vi "Build Blackboard Tag Table.vi"(8 "error in (no error)":errorcluster, 11 "Blackboard in":refnum<class "Blackboard.lvclass">) -> (0 "error out":errorcluster, 1 "Values":refnum<class "Abs_Value.lvclass">[](array[class]), 2 "Table":string[][](array[string]), 3 "Blackboard out":refnum<class "Blackboard.lvclass">)   [LabVIEW 2021]
uses:
  Blackboard/Blackboard.lvclass
  <vilib>/TSA/Abstract Data Classes/Abs_Types/Value/Abs_Value.lvclass
  <vilib>/TSA/Abstract Data Classes/Abs_Types/Integer/Abs_Integer.lvclass
  C:/Program Files (x86)/National Instruments/LabVIEW 2021/vi.lib/TSA/Abstract Data Classes/Abs_Types/Numeric/Abs_Numeric.lvclass
  C:/Program Files (x86)/National Instruments/LabVIEW 2021/vi.lib/TSA/Abstract Data Classes/Abs_Types/Value/Abs_Value.lvclass
  C:/Program Files (x86)/National Instruments/LabVIEW 2021/vi.lib/TSA/Abstract Data Classes/Abs_Types/Type/Abs_Type.lvclass
  C:/Program Files (x86)/National Instruments/LabVIEW 2021/vi.lib/TSA/Abstract Data Classes/Abs_Types/Integer/Abs_Integer.lvclass
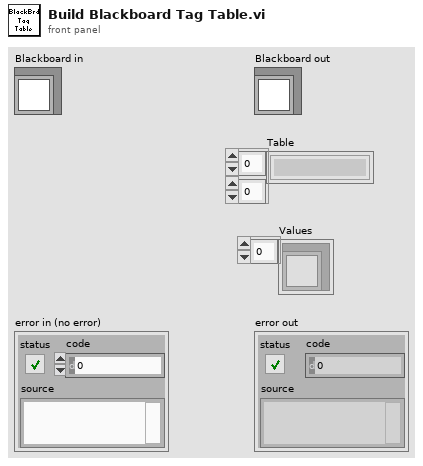
[diagram p1: front panel]
types:
  T1 = typedef "NI_Data Type.lvlib/Data Type.ctl" = enum8{"Invalid Type", "Void", "I8", "I16", "I32", "I64", "U8", "U16", "U32", "U64", "Single Float", "Double Float", "Extended Float", "Single Complex", "Double Complex", "Extended Complex", "Enum U8", "Enum U16", "Enum U32", "Enum U64", "Single Float With Unit", "Double Float With Unit", "Extended Float With Unit", "Single Complex with Unit", "Double Complex with Unit", "Extended Complex with Unit", "Boolean", "String", "Path", "Picture", "Tag", "Array", "Cluster", "Variant", "LV Variant", "Waveform", "Timestamp", "Digital Waveform", "Digital Data", "ExpressData", "Refnum", "External Data", "VI", "Poly VI", "LabVIEW Class Instance", "Fixed Point", "Set Collection", "Map Collection"}
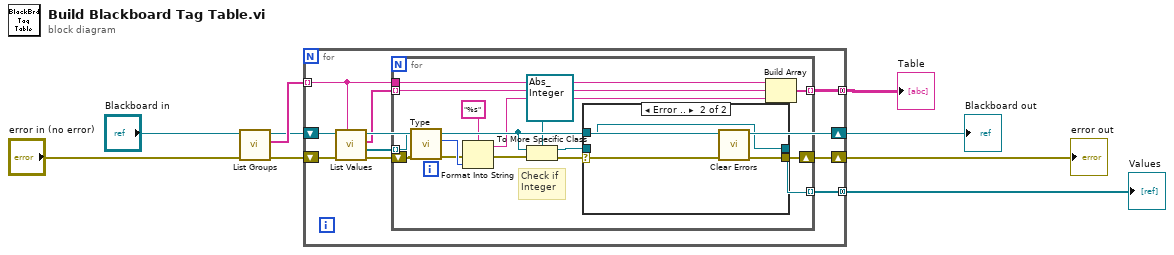
[diagram p0: block diagram]
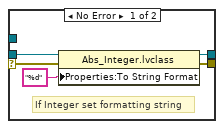
[diagram p2: hidden frame]
diagram:
  n1 = call "List Groups.vi"("error in (no error)"="error in (no error)", "Blackboard in"="Blackboard in") -> ("error out"=w6:errorcluster, "Groups"=w7:string[], "Blackboard out"=w4:refnum<class "Blackboard.lvclass">)  [unwired: 7 in]
  n2 = for {
    shift-right: [w19] -> w3
    shift-left: w4 -> [w18]
    shift-right: [w11] -> w2
    shift-left: w6 -> [w17]
    tunnel: w7 -> [w16] mode=indexing
    tunnel: [w14] -> w9 mode=concatenating
    tunnel: [w10] -> w1 mode=concatenating
    n3 = call "List Values.vi"("Group"=w16, "error in (no error)"=w17, "Blackboard in"=w18) -> ("error out"=w12:errorcluster, "Values"=w13:refnum<class "Abs_Value.lvclass">[], "Tags"=w15:string[], "Blackboard out"=w19:refnum<class "Blackboard.lvclass">)  [unwired: 5 in]
    n4 = for {
      tunnel: w16 -> [w35]
      tunnel: w15 -> [w34] mode=indexing
      tunnel: [w33] -> w14 mode=indexing
      tunnel: w13 -> [w31] mode=indexing
      shift-right: [w23] -> w11
      shift-left: w12 -> [w32]
      tunnel: [w27] -> w10 mode=indexing
      # "Check if\nInteger"
      n5 = call-dynamic "Type.vi"("error in (no error)"=w32, "Element in"=w31) -> ("error out"=w22:errorcluster, "Type"=w30:T1, "Element out"=w20:refnum<class "Abs_Value.lvclass">)  [unwired: 7 in]
      n6 = Format Into String(format string="%s", error in=w22, w30) -> (resulting string=w29:string, error out=w21:errorcluster)  [unwired: 1 in]
      n7 = To More Specific Class(target class=refnum<class "Abs_Integer.lvclass"> refnum ("Abs_Integer.lvclass"), reference=w20, error in=w21) -> (specific class reference=w25:refnum<class "Abs_Integer.lvclass">, error out=w26:errorcluster)
      n8 = case shown="Error .." w26 {
        selector: w26 -> [w39 w42]
        tunnel: [w40 w41] -> w27
        tunnel: w25 -> [w38 _]
        tunnel: [w36 w43] -> w23
        tunnel: w20 -> [_ w41]
        frame No Error {
          # "If Integer set formatting string"
          n9 = property class="Abs_Integer.lvclass"(reference=w38, error in=w39, "Properties:To String Format"="%d" ("To String Format")) -> (reference out=w40:refnum<class "Abs_Integer.lvclass">, error out=w36:errorcluster)
        }
        frame Error {
          n10 = call <vilib>:"Clear Errors.vi"("error in (no error)"=w42) -> ("error out"=w43:errorcluster)  [unwired: 5 in, 1 out]
        }
      }
      n11 = Build Array(w35, w34, w29) -> (w33:string[])
    }
  }
  "Table" <- w9
  "Blackboard out" <- w3
  "error out" <- w2
  "Values" <- w1
